vi "Generate_WayPoints_Hopping_IT_Surface_and_Bulk.vi"(11 "Input Cluster":T2={"Scan Rate (um/s)"=15.0, "X Start"=15.0, "X End"=15.0, "Y Start"=15.0, "Y End"=15.0, " Z Start"=15.0, "HoppingDistance"=1.0, "V"=15.0, "Z End"=15.0, "Approach Rate Hopping (um/s)"=15.0, "Retrack Rate (um/s)"=15.0, "V 1"=15.0, "HoldTime IT/s"=15.0, "HoldTime Bulk Pre IT/s 2"=15.0, "HoldTime Bulk IT Post/s"=15.0}) -> (0 "output cluster":T1)   [LabVIEW 2023]
uses:
  TypeDefs/WayPointCluster.ctl
panel:
  in  "WayPointCluster":T1
  out "Y  P":dbl
  out "X  P":dbl
  out "HoppingDistanceX":dbl
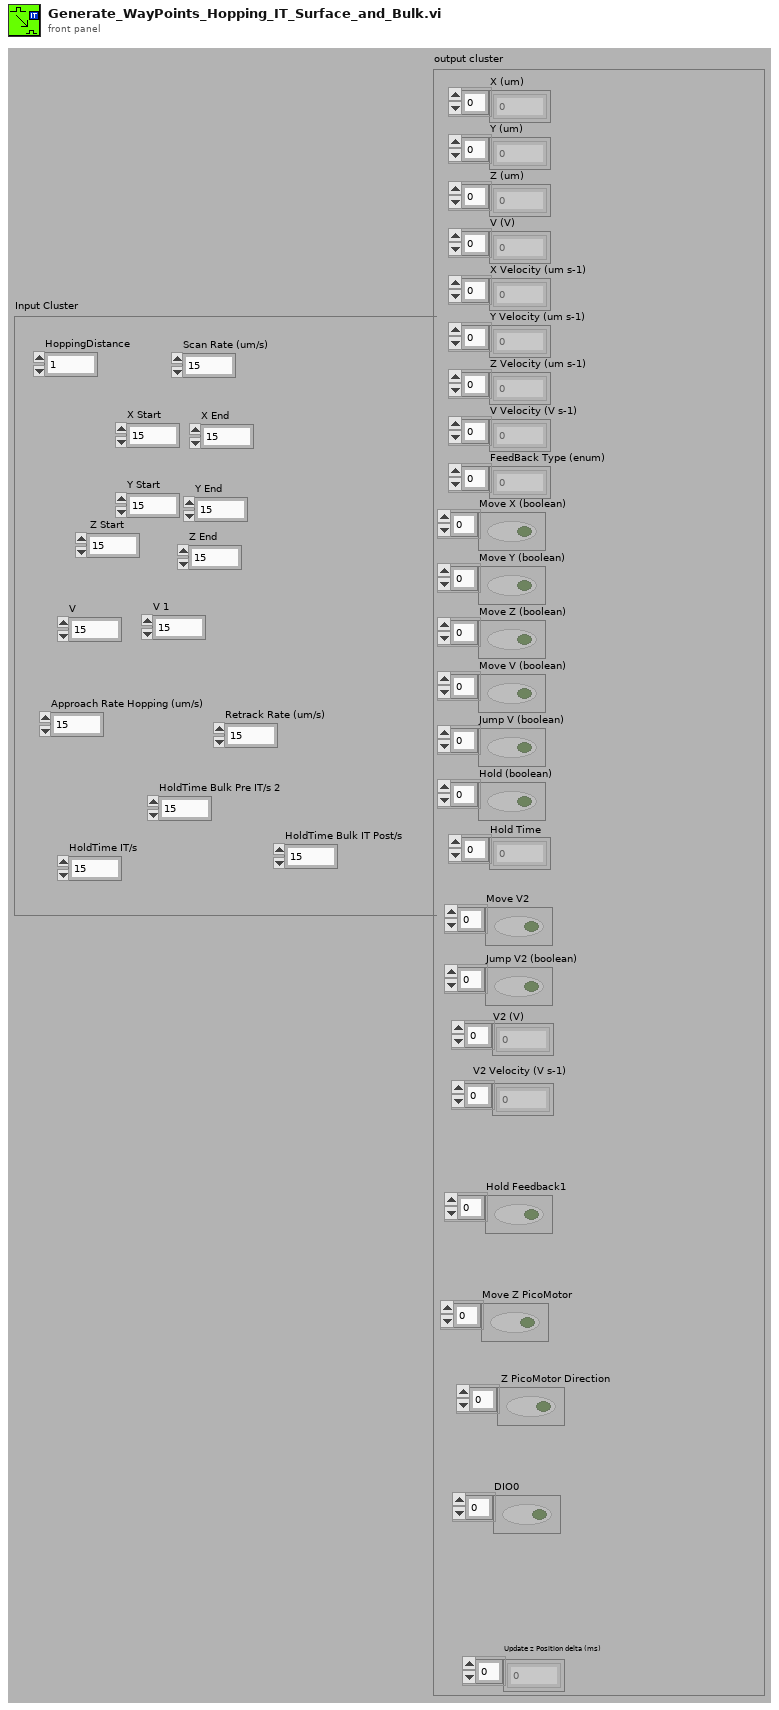
[diagram p1: front panel]
types:
  T1 = typedef "WayPointCluster.ctl" = cluster{"X (um)":dbl[], "Y (um)":dbl[], "Z (um)":dbl[], "V (V)":dbl[], "X Velocity (um s-1)":dbl[], "Y Velocity (um s-1)":dbl[], "Z Velocity (um s-1)":dbl[], "V Velocity (V s-1)":dbl[], "FeedBack Type (enum)":u16[], "Move X (boolean)":bool[], "Move Y (boolean)":bool[], "Move Z (boolean)":bool[], "Move V (boolean)":bool[], "Jump V (boolean)":bool[], "Hold (boolean)":bool[], "Hold Time":u32[], "V2 (V)":dbl[], "Move V2":bool[], "V2 Velocity (V s-1)":dbl[], "Jump V2 (boolean)":bool[], "Update z Position delta (ms)":i16[], "Hold Feedback1":bool[], "Move Z PicoMotor":bool[], " Z PicoMotor Direction":bool[], "DIO0":bool[]}
  T2 = cluster{"Scan Rate (um/s)":dbl, "X Start":dbl, "X End":dbl, "Y Start":dbl, "Y End":dbl, " Z Start":dbl, "HoppingDistance":dbl, "V":dbl, "Z End":dbl, "Approach Rate Hopping (um/s)":dbl, "Retrack Rate (um/s)":dbl, "V 1":dbl, "HoldTime IT/s":dbl, "HoldTime Bulk Pre IT/s 2":dbl, "HoldTime Bulk IT Post/s":dbl}
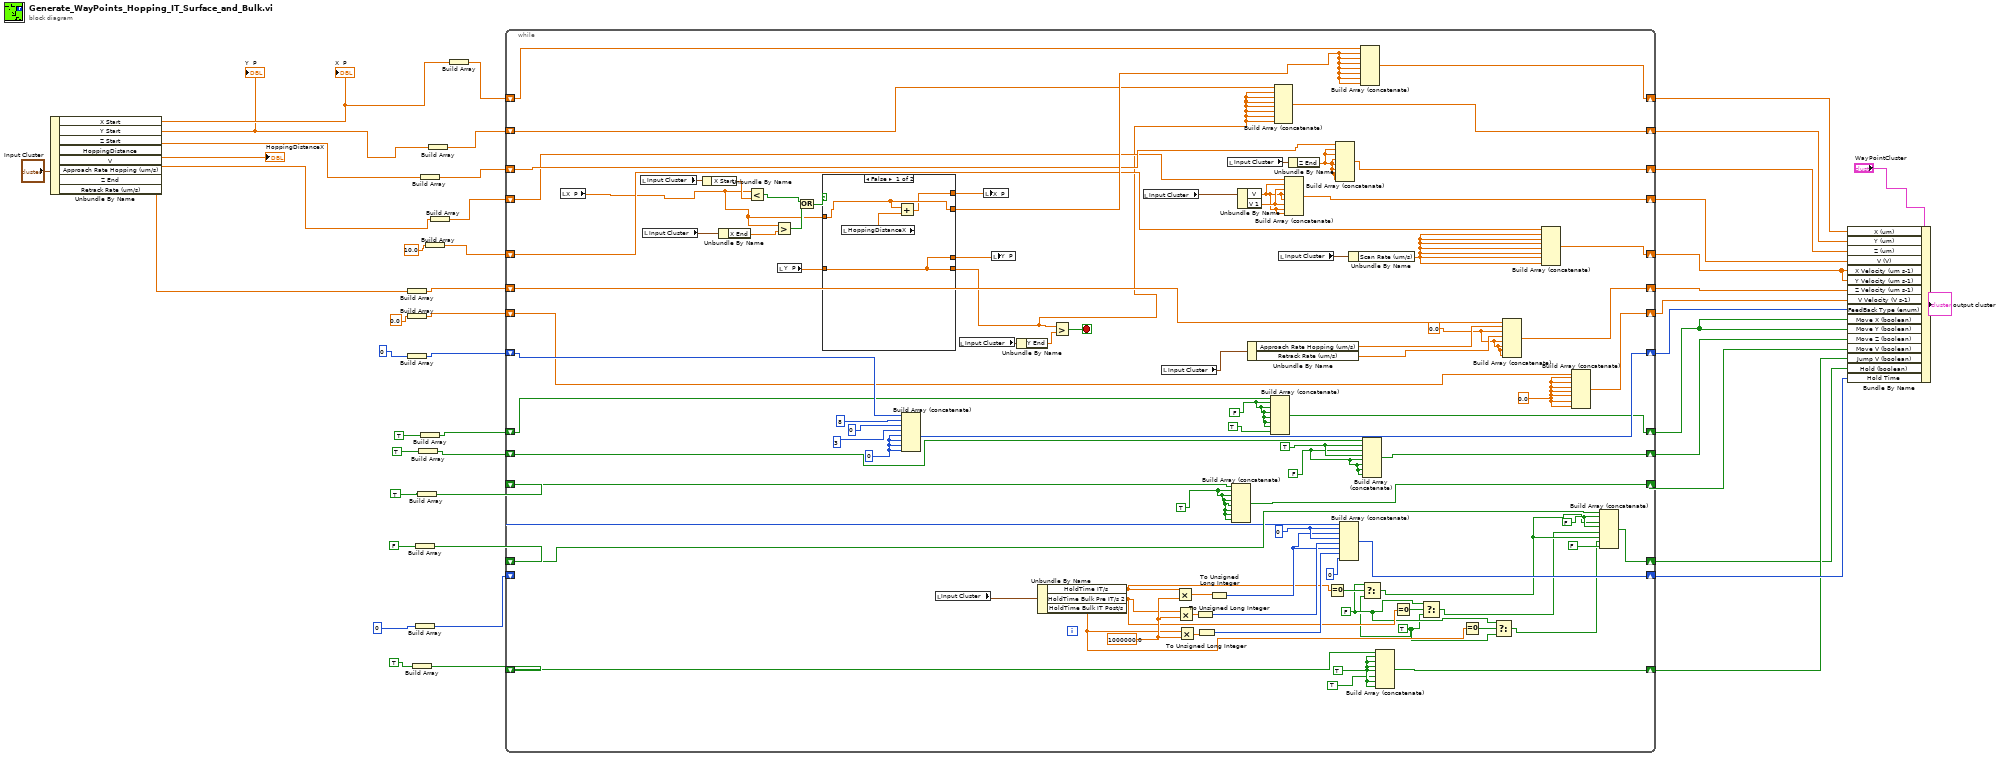
[diagram p0: block diagram]
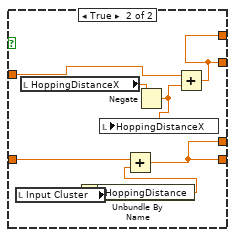
[diagram p2: hidden frame]
diagram:
  n1 = Unbundle By Name("Input Cluster") -> ("X Start"=w28:dbl, "Y Start"=w27:dbl, "Z Start"=w29:dbl, "HoppingDistance"=→"HoppingDistanceX":dbl, "V"=w26:dbl, "Approach Rate Hopping (um/s)"=w11:dbl)  [unwired: 2 out]
  "X  P" <- w28
  "Y  P" <- w27
  n2 = Build Array(w11) -> (w36:dbl[])
  n3 = Build Array(u16 0 ("element")) -> (w32:u16[])
  n4 = Build Array(0.0 ("element")) -> (w34:dbl[])
  n5 = Build Array(TRUE) -> (w21:bool[])
  n6 = Build Array(FALSE) -> (w14:bool[])
  n7 = Build Array(u32 0 ("element")) -> (w24:u32[])
  n8 = Build Array(TRUE) -> (w19:bool[])
  n9 = Build Array(TRUE) -> (w25:bool[])
  n10 = Build Array(w29) -> (w41:dbl[])
  n11 = Build Array(TRUE) -> (w2:bool[])
  n12 = Build Array(10.0 ("element")) -> (w37:dbl[])
  n13 = Build Array(w27) -> (w43:dbl[])
  n14 = Build Array(w26) -> (w39:dbl[])
  n15 = Build Array(w28) -> (w45:dbl[])
  n16 = while {
    shift-right: [w119] -> w44
    shift-left: w45 -> [w47]
    shift-right: [w116] -> w42
    shift-left: w43 -> [w117]
    shift-right: [w114] -> w40
    shift-left: w41 -> [w115]
    shift-right: [w111] -> w38
    shift-left: w39 -> [w91]
    shift-right: [w110] -> w4
    shift-left: w37 -> [w112]
    shift-right: [w108] -> w35
    shift-left: w36 -> [w109]
    shift-right: [w106] -> w33
    shift-left: w34 -> [w107]
    shift-right: [w133] -> w31
    shift-left: w32 -> [w134]
    shift-right: [w104] -> w23
    shift-left: w25 -> [w105]
    shift-right: [w99] -> w7
    shift-left: w14 -> [w100]
    shift-right: [w97] -> w22
    shift-left: w24 -> [w98]
    shift-right: [w94] -> w20
    shift-left: w21 -> [w95]
    shift-right: [w102] -> w6
    shift-left: w19 -> [w103]
    shift-right: [w72] -> w1
    shift-left: w2 -> [w75]
    stop <- w88 stop-if-true
    w48 = TRUE
    w49 = FALSE
    w73 = FALSE
    w76 = 0.0 ("element")
    w83 = u16 0 ("element")
    w65 = 1000000.0 ("element")
    w93 = TRUE
    w101 = TRUE
    w66 = u32 0 ("element")
    w69 = FALSE
    w70 = FALSE
    w71 = TRUE
    w77 = 0.0 ("element")
    n17 = local read "X  P"() -> (w89:dbl)
    n18 = local read "Input Cluster"() -> (w136:T2)
    n19 = local read "Input Cluster"() -> (w135:T2)
    n20 = Unbundle By Name(w136) -> ("X Start"=w130:dbl)
    n21 = Unbundle By Name(w135) -> ("X End"=w128:dbl)
    n22 = Less?(x=w89, y=w130) -> (x < y?=w129:bool)
    n23 = Greater?(x=w89, y=w128) -> (0:w127:bool)
    n24 = local read "Y  P"() -> (w123:dbl)
    n25 = Or(x=w129, y=w127) -> (x .or. y?=w126:bool)
    n26 = case shown="False" w126 {
      tunnel: [w138 w141] -> w118
      tunnel: w89 -> [w138 w142]
      tunnel: w123 -> [w140 w145]
      tunnel: [w140 w144] -> w87
      tunnel: [w140 w144] -> w122
      tunnel: [w137 w141] -> w121
      frame False {
        n27 = local read "HoppingDistanceX"() -> (w139:dbl)
        n28 = Add(x=w138, y=w139) -> (x+y=w137:dbl)
      }
      frame True {
        n29 = local read "Input Cluster"() -> (w147:T2)
        n30 = local read "HoppingDistanceX"() -> (w148:dbl)
        n31 = Unbundle By Name(w147) -> ("HoppingDistance"=w146:dbl)
        n32 = Add(x=w145, y=w146) -> (x+y=w144:dbl)
        n33 = Negate(x=w148) -> (-x=w143:dbl)
        n34 = local write "HoppingDistanceX"(w143) -> ()
        n35 = Add(x=w142, y=w143) -> (x+y=w141:dbl)
      }
    }
    n36 = Build Array (concatenate)(w134, u16 8 ("element"), u16 0 ("element"), u16 3 ("element"), w83, w83, w83, w83) -> (w133:u16[])
    n37 = local read "Input Cluster"() -> (w96:T2)
    n38 = local read "Input Cluster"() -> (w125:T2)
    n39 = local write "X  P"(w121) -> ()
    n40 = local write "Y  P"(w122) -> ()
    n41 = Unbundle By Name(w125) -> ("Y End"=w124:dbl)
    n42 = Unbundle By Name(w96) -> ("HoldTime IT/s"=w58:dbl, "HoldTime Bulk Pre IT/s 2"=w57:dbl, "HoldTime Bulk IT Post/s"=w56:dbl)
    n43 = Greater?(x=w87, y=w124) -> (0:w88:bool)
    n44 = local read "Input Cluster"() -> (w131:T2)
    n45 = local read "Input Cluster"() -> (w120:T2)
    n46 = Multiply(x=w58, y=w65) -> (x*y=w67:dbl)
    n47 = Multiply(x=w57, y=w65) -> (x*y=w64:dbl)
    n48 = Multiply(x=w56, y=w65) -> (x*y=w63:dbl)
    n49 = To Unsigned Long Integer(number=w64) -> (unsigned 32bit integer=w62:u32)
    n50 = To Unsigned Long Integer(number=w63) -> (unsigned 32bit integer=w60:u32)
    n51 = To Unsigned Long Integer(number=w67) -> (unsigned 32bit integer=w61:u32)
    n52 = local read "Input Cluster"() -> (w132:T2)
    n53 = Build Array (concatenate)(w103, w101, w101, w101, w101, w101, w101, w101) -> (w102:bool[])
    n54 = Unbundle By Name(w131) -> ("V"=w81:dbl, "V 1"=w82:dbl)
    n55 = Unbundle By Name(w120) -> ("Approach Rate Hopping (um/s)"=w79:dbl, "Retrack Rate (um/s)"=w78:dbl)
    n56 = Build Array (concatenate)(w75, w73, w73, w73, w73, w73, w73, TRUE) -> (w72:bool[])
    n57 = Build Array (concatenate)(w117, w87, w87, w87, w87, w87, w87, w87) -> (w116:dbl[])
    n58 = local read "Input Cluster"() -> (w90:T2)
    n59 = Build Array (concatenate)(w91, w81, w82, w81, w81, w82, w81, w81) -> (w111:dbl[])
    n60 = Unbundle By Name(w132) -> ("Z End"=w113:dbl)
    n61 = Equal To 0?(x=w58) -> (x = 0?=w53:bool)
    n62 = Build Array (concatenate)(w115, w113, w113, w113, w113, w113, w113, w113) -> (w114:dbl[])
    n63 = Build Array (concatenate)(w98, w66, w61, w66, w62, w61, w60, u32 0 ("element")) -> (w97:u32[])
    n64 = Unbundle By Name(w90) -> ("Scan Rate (um/s)"=w80:dbl)
    n65 = Build Array (concatenate)(w47, w118, w118, w118, w118, w118, w118, w118) -> (w119:dbl[])
    n66 = Build Array (concatenate)(w105, w71, w70, w71, w70, w70, w70, w70) -> (w104:bool[])
    n67 = Select(t=w49, s=w53, f=w48) -> (s? t:f=w52:bool)
    n68 = Build Array (concatenate)(w95, w93, w93, w93, w93, TRUE, w93, w93) -> (w94:bool[])
    n69 = Equal To 0?(x=w57) -> (x = 0?=w54:bool)
    n70 = Select(t=w49, s=w54, f=w48) -> (s? t:f=w51:bool)
    n71 = Equal To 0?(x=w56) -> (x = 0?=w55:bool)
    n72 = Select(t=w49, s=w55, f=w48) -> (s? t:f=w50:bool)
    n73 = Build Array (concatenate)(w109, w79, w77, w78, w77, w77, w77, w77) -> (w108:dbl[])
    n74 = Build Array (concatenate)(w112, w80, w80, w80, w80, w80, w80, w80) -> (w110:dbl[])
    n75 = Build Array (concatenate)(w107, w76, w76, w76, w76, w76, w76, w76) -> (w106:dbl[])
    n76 = Build Array (concatenate)(w100, w69, w52, w69, w51, w52, w50, FALSE) -> (w99:bool[])
  }
  n77 = Bundle By Name(cluster="WayPointCluster", "X (um)"=w44, "Y (um)"=w42, "Z (um)"=w40, "V (V)"=w38, "X Velocity (um s-1)"=w4, "Y Velocity (um s-1)"=w4, "Z Velocity (um s-1)"=w35, "V Velocity (V s-1)"=w33, "FeedBack Type (enum)"=w31, "Move X (boolean)"=w1, "Move Y (boolean)"=w1, "Move Z (boolean)"=w23, "Move V (boolean)"=w6, "Jump V (boolean)"=w20, "Hold (boolean)"=w7, "Hold Time"=w22) -> (→"output cluster":T1)
